vi "Add Library Icon Layer.vi"(8 "error in (no error)":errorcluster, 11 "VI Ref":refnum<vi>) -> (0 "error out":errorcluster, 2 "Save?":bool, 3 "VI Ref out":refnum<vi>)   [LabVIEW 2020, in "Code Cleanup.lvlib"]
uses:
  Code Cleanup.lvlib
  <vilib>/LabVIEW Icon API/lv_icon/Classes/Layer/Layer.lvclass
  <vilib>/LabVIEW Icon API/lv_icon/Classes/Icon/Icon.lvclass
  <vilib>/LabVIEW Icon API/LabVIEW Icon API.lvlib
  <vilib>/LabVIEW Icon API/lv_icon/Controls/LayerType.ctl
  <vilib>/LabVIEW Icon API/lv_icon/Controls/Graphic.ctl
  <vilib>/LabVIEW Icon API/lv_icon/Classes/Icon Framework/Icon Framework.lvclass
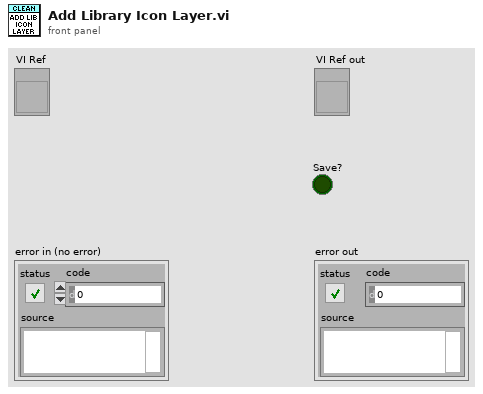
[diagram p1: front panel]
types:
  T1 = typedef "LayerType.ctl" = enum16{"Graphic", "Text", "Tool", "Graphic Drop"}
  T2 = typedef "Layer.ctl" = cluster{"LayerIcon":picture, "LayerName":string, "Opacity":u8, "Visibility?":bool}
  T3 = typedef "Graphic.ctl" = cluster{"Rectangle":cluster{"left":i16, "top":i16, "right":i16, "bottom":i16}, "Path":path, "Image":picture, "Filter":string, "FileName":string}
  T4 = typedef "BodyText.ctl" = cluster{"Line 1 text":string, "Line 2 text":string, "Line 3 text":string, "Line 4 text":string, "Line 1 color":u32, "Line 2 color":u32, "Line 3 color":u32, "Line 4 color":u32, "Body Text Spec":cluster{"Font":T5, "Alignment":T6, "Size":u8}, "Center text vertically":bool, "Capitalize Text":bool}
  T5 = typedef "Font.ctl" = string
  T6 = typedef "Alignment.ctl" = u16
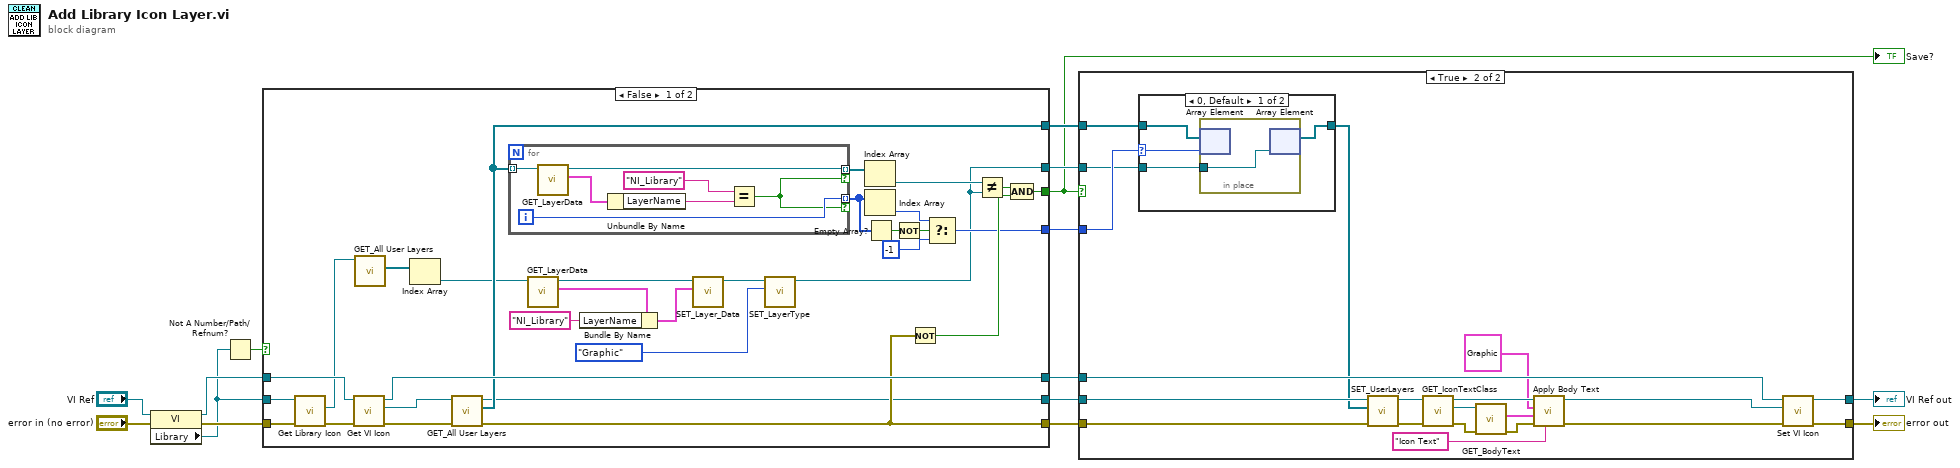
[diagram p0: block diagram]
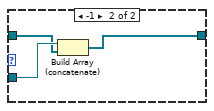
[diagram p4: hidden frame]
diagram:
  n1 = property class="VI"(reference="VI Ref", error in="error in (no error)") -> (reference out=w8:refnum<vi>, error out=w9:errorcluster, "Library"=w5:refnum<vi>)
  n2 = Not A Number/Path/Refnum?(number/path/refnum=w5) -> (NaN/Path/Refnum?=w4:bool)
  n3 = case shown="False" w4 {
    tunnel: [w45 w55] -> w14
    tunnel: [w44 _] -> w13
    tunnel: [w43 w54] -> w12
    tunnel: [w42 _] -> w11
    tunnel: w9 -> [w39 w54]
    tunnel: w8 -> [w37 w55]
    tunnel: [w16 _] -> w7
    tunnel: [w17 _] -> w6
    tunnel: [w24 _] -> w3
    tunnel: w5 -> [w23 _]
    frame False {
      n4 = call <vilib>:"Get Library Icon.vi"("error in (no error)"=w39, "Library Refnum in"=w23) -> ("error out"=w38:errorcluster, "Icon"=w36:refnum<class "Icon.lvclass">)  [unwired: 7 in, 1 out]
      n5 = call <vilib>:"Get VI Icon.vi"("error in (no error)"=w38, "VI Refnum in"=w37) -> ("error out"=w41:errorcluster, "Icon"=w40:refnum<class "Icon.lvclass">, "VI Refnum out"=w45:refnum<vi>)  [unwired: 7 in]
      n6 = call-dynamic "GET_All User Layers.vi"("Icon.lvclass in"=w36) -> ("User Layer"=w35:refnum<class "Layer.lvclass">[])  [unwired: 8 in, 2 out]
      n7 = Index Array(array=w35) -> (element=w34:refnum<class "Layer.lvclass">)  [unwired: 1 in]
      n8 = call-dynamic "GET_All User Layers.vi"("error in (no error)"=w41, "Icon.lvclass in"=w40) -> ("error out"=w43:errorcluster, "User Layer"=w44:refnum<class "Layer.lvclass">[], "Icon.lvclass out"=w42:refnum<class "Icon.lvclass">)  [unwired: 7 in]
      n9 = for {
        tunnel: w44 -> [w52] mode=indexing
        tunnel: [w49] -> w33 mode=indexing if=w47
        tunnel: [w48] -> w22 mode=indexing if=w47
        i -> [w48]
        n10 = call-dynamic "GET_LayerData.vi"("Layer.lvclass in"=w52) -> ("Data"=w53:T2, "Layer.lvclass out"=w49:refnum<class "Layer.lvclass">)  [unwired: 6 in, 3 out]
        n11 = Unbundle By Name(w53) -> ("LayerName"=w51:string)
        n12 = Equal?(x="NI_Library", y=w51) -> (x = y?=w47:bool)
      }
      n13 = call-dynamic "GET_LayerData.vi"("Layer.lvclass in"=w34) -> ("Data"=w30:T2, "Layer.lvclass out"=w27:refnum<class "Layer.lvclass">)  [unwired: 6 in, 3 out]
      n14 = Bundle By Name(cluster=w30, "LayerName"="NI_Library") -> (w28:T2)
      n15 = call-dynamic "SET_Layer_Data.vi"("Data"=w28, "Layer.lvclass in"=w27) -> ("Layer.lvclass out"=w26:refnum<class "Layer.lvclass">)  [unwired: 8 in, 1 out]
      n16 = call-dynamic "SET_LayerType.vi"("Type"=LayerType."Graphic", "Layer.lvclass in"=w26) -> ("Layer.lvclass out"=w16:refnum<class "Layer.lvclass">)  [unwired: 8 in, 1 out]
      n17 = Index Array(array=w33) -> (element=w32:refnum<class "Layer.lvclass">)  [unwired: 1 in]
      n18 = Index Array(array=w22) -> (element=w19:i32)  [unwired: 1 in]
      n19 = Empty Array?(array=w22) -> (empty?=w21:bool)
      n20 = Not(x=w21) -> (.not. x?=w20:bool)
      n21 = Not(x=w43) -> (.not. x?=w46:bool)
      n22 = Select(t=w19, s=w20, f=-1) -> (s? t:f=w17:i32)
      n23 = Not Equal?(x=w32, y=w16) -> (x != y?=w31:bool)
      n24 = Compound Arithmetic op=AND(w31, w46) -> (w24:bool)
    }
    frame True {
    }
  }
  "Save?" <- w3
  n25 = case shown="True" w3 {
    tunnel: w12 -> [w57 w77]
    tunnel: [w57 w74] -> w15
    tunnel: [w56 w73] -> w10
    tunnel: w14 -> [w56 w75]
    tunnel: w13 -> [_ w71]
    tunnel: w7 -> [_ w70]
    tunnel: w11 -> [_ w76]
    tunnel: w6 -> [_ w72]
    frame False {
    }
    frame True {
      n26 = case shown="0, Default" w72 {
        selector: w72 -> [w80 _]
        tunnel: w71 -> [w81 w84]
        tunnel: w70 -> [w79 w85]
        tunnel: [w78 w83] -> w69
        frame 0, Default {
          n27 = in-place {
            in-place-border: w79 -> [w82]
            n28 = in-place-array #1(w81, w80) -> ()  [unwired: 1 out]
            n29 = in-place-array #1(w82) -> (w78:refnum<class "Layer.lvclass">[])  [unwired: 1 out]
          }
        }
        frame -1 {
          n30 = Build Array (concatenate)(w85, w84) -> (w83:refnum<class "Layer.lvclass">[])
        }
      }
      n31 = call-dynamic "SET_UserLayers.vi"("error in (no error)"=w77, "Layers"=w69, "Icon.lvclass in"=w76) -> ("error out"=w67:errorcluster, "Icon.lvclass out"=w68:refnum<class "Icon.lvclass">)  [unwired: 7 in]
      n32 = call-dynamic "GET_IconTextClass.vi"("error in (no error)"=w67, "Icon.lvclass in"=w68) -> ("error out"=w66:errorcluster, "Icon Framework.lvclass"=w65:refnum<class "Icon Framework.lvclass">, "Icon.lvclass out"=w64:refnum<class "Icon.lvclass">)  [unwired: 7 in]
      n33 = call-dynamic "GET_BodyText.vi"("error in (no error)"=w66, "Icon Framework.lvclass in"=w65) -> ("error out"=w61:errorcluster, "Body Text"=w62:T4)  [unwired: 6 in, 2 out]
      n34 = call <vilib>:"Apply Body Text.vi"("Layer name"="Icon Text", "error in (no error)"=w61, "Body test"=w62, "Path & Icon"=T3 {"Rectangle"={"left"=0, "top"=0, "right"=0, "bottom"=0}, "Path"=path "", "Image"=bytes[0], "Filter"="", "FileName"=""} ("Path and Icon Template"), "Icon in"=w64) -> ("error out"=w59:errorcluster, "Icon out"=w58:refnum<class "Icon.lvclass">)  [unwired: 4 in, 1 out]
      n35 = call <vilib>:"Set VI Icon.vi"("error in (no error)"=w59, "Icon"=w58, "VI Refnum in"=w75) -> ("error out"=w74:errorcluster, "VI Refnum out"=w73:refnum<vi>)  [unwired: 7 in]
    }
  }
  "error out" <- w15
  "VI Ref out" <- w10
